vi "Set Process Event Registration.vi"(8 "error in (no error)":errorcluster, 10 "Event Registration Refnum":T1, 11 "SMO in":refnum<class "SMO.lvclass">) -> (0 "error out":errorcluster, 3 "SMO out":refnum<class "SMO.lvclass">)   [LabVIEW 2021, in "smo.lvlib" / "SMO.lvclass"]
uses:
  SMO.lvclass
  Typedefs/ProcessRegistrationRefnum.ctl
  Typedefs/SMOState --Enum.ctl
  Typedefs/AbortProcessEventData--Cluster.ctl
  Typedefs/StopProcessEventData--Cluster.ctl
  Typedefs/SMO Dependency Event--Cluster.ctl
  Typedefs/SMO Dependency Event--Enum.ctl
  Support/Attribute.Owner/Packet -- Cluster.ctl
  SMO.lvclass/SMO.ctl
  Support/Attribute.Owner/Attribute.Owner.lvclass
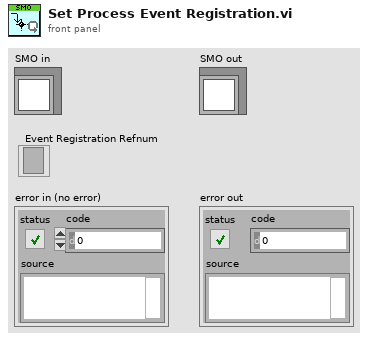
[diagram p1: front panel]
types:
  T1 = typedef "smo.lvlib/SMO.lvclass/ProcessRegistrationRefnum.ctl" = refnum<event-registration>
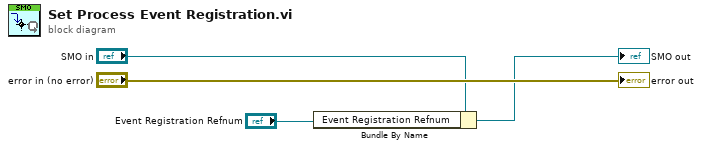
[diagram p0: block diagram]
diagram:
  n1 = Bundle By Name(cluster="SMO in", "Event Registration Refnum"="Event Registration Refnum") -> (→"SMO out":refnum<class "SMO.lvclass">)
  "error out" <- "error in (no error)"
